vi "GA_Main_ini.vi"() -> ()   [LabVIEW 2018]
uses:
  3306bcb4-fbbd-4c65-bae6-1e6ebe767a75.vi
  GA_Global.vi
panel:
  out "pop(500*20)":i32[][](array[numeric])
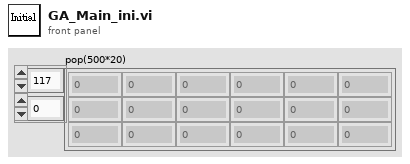
[diagram p1: front panel]
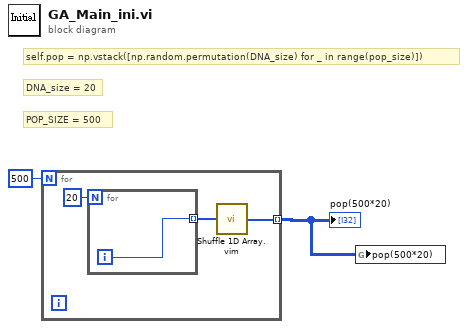
[diagram p0: block diagram]
diagram:
  # "POP_SIZE = 500"
  # "DNA_size = 20"
  # "self.pop = np.vstack([np.random.permutation(DNA_size) for _ in range(pop_size)])"
  n1 = for {
    N: 500 -> [_]
    tunnel: [w3] -> w1 mode=indexing
    n2 = for {
      N: 20 -> [_]
      tunnel: [w6] -> w4 mode=indexing
      i -> [w6]
    }
    n3 = call "Shuffle 1D Array.vim"("array"=w4) -> ("shuffled array"=w3:i32[])  [unwired: 4 in]
  }
  "pop(500*20)" <- w1
  n4 = global write "GA_Global.vi" "pop(500*20)"(w1) -> ()
